vi "Dictionary Update (by value)__ogtk.vi"(7 "unlock dictionary? (FALSE)":bool, 8 "error in (no error)":errorcluster, 10 "dictionary with updates":T1[](array[typedef]), 11 "dictionary":T2) -> (0 "error out":errorcluster, 2 "created new?":bool[](array[boolean]), 3 "dictionary out":T2)   [LabVIEW 2011]
doc: "Looks for all the keys and writes the respective values to the dictionary linked to specified dictionary reference.\n\n<B>unlock dictionary</B> will unlock a previously locked dictionary. Locking a dictionary is useful when the values of keys store compound data, which might be modified in multiple locations."
uses:
  Dictionary Object RefNum__ogtk.ctl
  Dictionary Object RefNum - Enum__ogtk.ctl
  Dictionary Key Value Pair Cluster__ogtk.ctl
panel:
  # "Dictionary Update (by value).vi\n\nLooks for all the keys and writes the respective values to the dictionary linked to specified dictionary reference.\n\nPlease visit http://www.OpenG.org to learn about the\nOpen Source LabVIEW software movement.\n\nNOTICE -- YOU MUST LEAVE THIS NOTICE IN PLACE.  PER THE TERMS OF THE LICENSE BELOW, YOU MAY SUBLICENSE THIS SOFTWARE \nIN ANY WAY THAT DOES NOT CONFLICT WITH THIS LICENSE.\n\n### BSD License (http://www.opensource.org/licenses/bsd-license.php) Begin ###\n \nCopyright (c) 2005, Jim Kring <jim@jimkring.com>\n\nAll rights reserved.\n\nRedistribution and use in source and binary forms, with or without modification, are permitted provided that the following conditions are met:\n\n    * Redistributions of source code must retain the above copyright notice, this list of conditions and the following disclaimer.\n    * Redistributions in binary form must reproduce the above copyright notice, this list of conditions and the following disclaimer in the \n       documentation and/or other materials provided with the distribution.\n    * Neither the name of SciWare, James Kring, Inc., nor the names of its contributors may be used to endorse or promote products derived \n       from this software without specific prior written permission.\n\nTHIS SOFTWARE IS PROVIDED BY THE COPYRIGHT HOLDERS AND CONTRIBUTORS \"AS IS\" AND ANY EXPRESS OR IMPLIED WARRANTIES, \nINCLUDING, BUT NOT LIMITED TO, THE IMPLIED WARRANTIES OF MERCHANTABILITY AND FITNESS FOR A PARTICULAR PURPOSE ARE \nDISCLAIMED. IN NO EVENT SHALL THE COPYRIGHT OWNER OR CONTRIBUTORS BE LIABLE FOR ANY DIRECT, INDIRECT, INCIDENTAL,\n SPECIAL, EXEMPLARY, OR CONSEQUENTIAL DAMAGES (INCLUDING, BUT NOT LIMITED TO, PROCUREMENT OF SUBSTITUTE GOODS OR \nSERVICES; LOSS OF USE, DATA, OR PROFITS; OR BUSINESS INTERRUPTION) HOWEVER CAUSED AND ON ANY THEORY OF LIABILITY, \nWHETHER IN CONTRACT, STRICT LIABILITY, OR TORT (INCLUDING NEGLIGENCE OR OTHERWISE) ARISING IN ANY WAY OUT OF THE USE \nOF THIS SOFTWARE, EVEN IF ADVISED OF THE POSSIBILITY OF SUCH DAMAGE.\n\n### BSD License End ###"
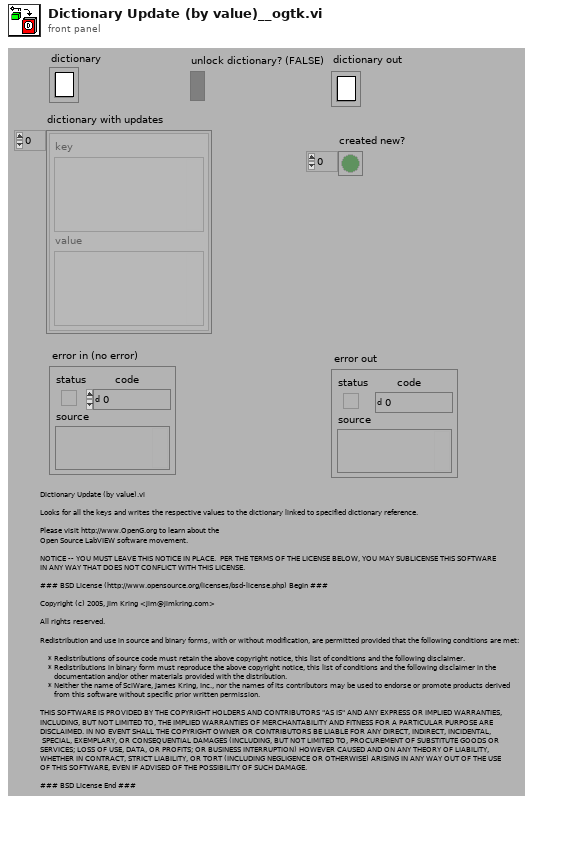
[diagram p1: front panel]
types:
  T1 = typedef "Dictionary Key Value Pair Cluster__ogtk.ctl" = cluster{"key":variant, "value":variant}
  T2 = typedef "Dictionary Object RefNum__ogtk.ctl" = refnum<k1>
  T3 = typedef "Dictionary Data__ogtk.ctl" = cluster{"keys":variant[], "values":variant[]}
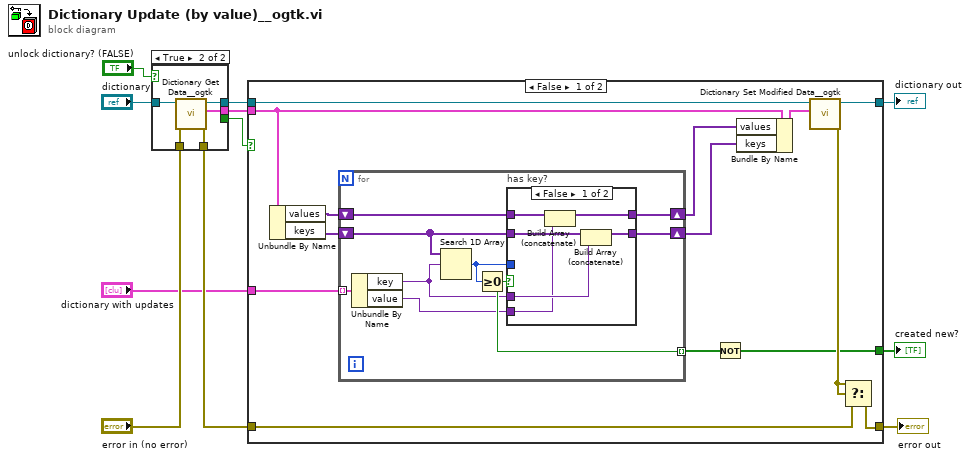
[diagram p0: block diagram]
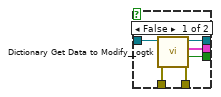
[diagram p2: hidden frame]
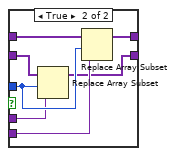
[diagram p3: hidden frame]
diagram:
  n1 = case shown="True" "unlock dictionary? (FALSE)" {
    tunnel: "error in (no error)" -> [w17 w22]
    tunnel: [w16 w21] -> w9
    tunnel: [w15 w20] -> w8
    tunnel: [w14 _] -> w7
    tunnel: "dictionary" -> [w13 w19]
    tunnel: [w12 w18] -> w4
    frame False {
      n2 = call "Dictionary Get Data to Modify__ogtk.vi"("error in (no error)"=w17, "Object RefNum"=w13) -> ("error out"=w15:errorcluster, "timed out"=w14:bool, "Data out"=w16:T3, "Dup Object RefNum"=w12:T2)  [unwired: 6 in]
    }
    frame True {
      n3 = call "Dictionary Get Data__ogtk.vi"("error in (no error)"=w22, "Object RefNum"=w19) -> ("error out"=w20:errorcluster, "Data out"=w21:T3, "Dup Object RefNum"=w18:T2)  [unwired: 7 in]
    }
  }
  n4 = case shown="False" w7 {
    tunnel: w9 -> [w35 _]
    tunnel: w8 -> [w31 w60]
    tunnel: [w30 w60] -> w10
    tunnel: [w34 w59] -> w5
    tunnel: w4 -> [w33 w59]
    tunnel: "dictionary with updates" -> [w29 _]
    tunnel: [w23 _] -> w2
    frame False {
      n5 = Unbundle By Name(w35) -> ("values"=w27:variant[], "keys"=w28:variant[])
      n6 = for {
        tunnel: w29 -> [w45] mode=indexing
        shift-right: [w38] -> w26
        shift-left: w27 -> [w39]
        shift-right: [w37] -> w25
        shift-left: w28 -> [w40]
        tunnel: [w43] -> w24 mode=indexing
        n7 = Unbundle By Name(w45) -> ("key"=w42:variant, "value"=w41:variant)
        n8 = Search 1D Array(1D array=w40, element=w42) -> (index of element=w44:i32)  [unwired: 1 in]
        n9 = Greater Or Equal To 0?(x=w44) -> (x >= 0?=w43:bool)
        n10 = case "has key?" shown="False" w43 {
          tunnel: w44 -> [_ w56]
          tunnel: w39 -> [w51 w58]
          tunnel: w40 -> [w50 w57]
          tunnel: w42 -> [w47 w55]
          tunnel: w41 -> [w46 w54]
          tunnel: [w49 w53] -> w37
          tunnel: [w48 w52] -> w38
          frame False {
            n11 = Build Array (concatenate)(w51, w46) -> (w48:variant[])
            n12 = Build Array (concatenate)(w50, w47) -> (w49:variant[])
          }
          frame True {
            n13 = Replace Array Subset(array=w57, new element=w55, index=w56) -> (w53:variant[])
            n14 = Replace Array Subset(array=w58, new element=w54, index=w56) -> (w52:variant[])
          }
        }
      }
      n15 = Not(x=w24) -> (.not. x?=w23:bool[])
      n16 = Bundle By Name(cluster=w35, "values"=w26, "keys"=w25) -> (w36:T3)
      n17 = call "Dictionary Set Modified Data__ogtk.vi"("Data in"=w36, "Object RefNum"=w33) -> ("error out"=w32:errorcluster, "dup Object RefNum"=w34:T2)  [unwired: 8 in]
      n18 = Select(t=w32, s=w32, f=w31) -> (s? t:f=w30:errorcluster)
    }
    frame True {
      # "Error or timed out"
    }
  }
  "error out" <- w10
  "dictionary out" <- w5
  "created new?" <- w2
